vi "DBL Angle to U16.vi"(10 "angle to u16 scale factor":dbl, 11 "Desired angle (degrees)":dbl min=0.0 format="%#_f") -> (2 "Actual angle (degrees)":dbl min=0.0 format="%#_f", 3 "u16":u16)   [LabVIEW 2013, in "Engine Simulation Toolkit System Explorer.lvlib"]
uses:
  Engine Simulation Toolkit System Explorer.lvlib
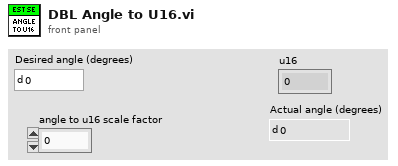
[diagram p1: front panel]
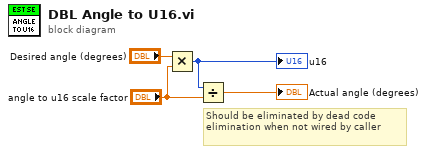
[diagram p0: block diagram]
diagram:
  # "Should be eliminated by dead code elimination when not wired by caller"
  n1 = Multiply(x="Desired angle (degrees)", y="angle to u16 scale factor") -> (x*y=w2:u16)
  "u16" <- w2
  n2 = Divide(x=w2, y="angle to u16 scale factor") -> (x/y=→"Actual angle (degrees)":dbl)
